vi "Get_FPGASimIO_Trigger Data_5734.vi"(7 "Channel Name":string="Trig0", 8 "Error In":errorcluster) -> (0 "Error Out":errorcluster, 3 "Trig Data":bool)   [LabVIEW 2012]
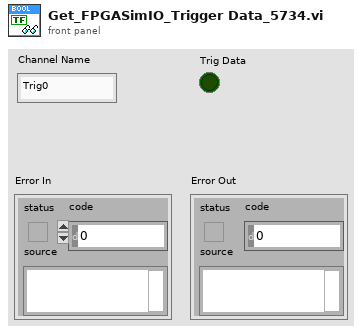
[diagram p1: front panel]
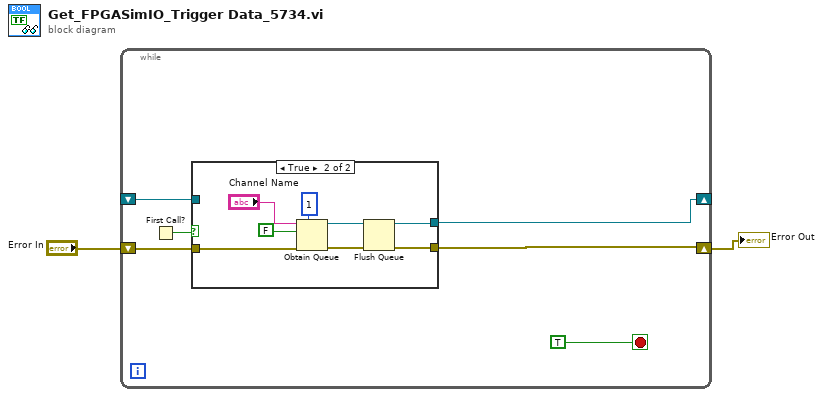
[diagram p0: block diagram]
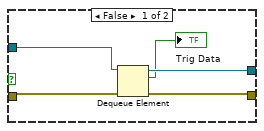
[diagram p2: hidden frame]
diagram:
  n1 = while {
    shift-right: [w3] -> w1
    shift-left: "Error In" -> [w7]
    shift-right: [w4] -> _
    shift-left: _ -> [w5]
    stop <- TRUE ("stop") stop-if-true
    n2 = First Call?() -> (First Call?: T/F=w8:bool)
    n3 = case shown="True" w8 {
      tunnel: [w11 w16] -> w4
      tunnel: [w12 w14] -> w3
      tunnel: w5 -> [w10 _]
      tunnel: w7 -> [w13 w20]
      frame False {
        n4 = Dequeue Element(queue=w10, error in (no error)=w13) -> (queue out=w11:refnum<queue>, element=→"Trig Data":bool, error out=w12:errorcluster)  [unwired: 1 in, 1 out]
      }
      frame True {
        n5 = Obtain Queue(max queue size (-1, unlimited)=1, name (unnamed)="Channel Name", element data type=FALSE, error in (no error)=w20) -> (queue out=w19:refnum<queue>, error out=w15:errorcluster)  [unwired: 1 in, 1 out]
        n6 = Flush Queue(queue=w19, error in (no error)=w15) -> (queue out=w16:refnum<queue>, error out=w14:errorcluster)  [unwired: 1 out]
      }
    }
  }
  "Error Out" <- w1
